vi "Append Element(s) to Dataset (Variant).vi"(4 "Data Element(s)":variant, 6 "error in (no error)":errorcluster, 8 "Dimension to Extend (0)":i32, 9 "HDF5 Dataset Ref":T1) -> (0 "error out":errorcluster, 1 "Number of Elements Added":i32, 2 "First Element Index":u64[](array[numeric]), 3 "HDF5 Dataset out":T1)   [LabVIEW 2017]
doc: "Appends one or more elements to an unlimited dataset."
uses:
  <vilib>/UPVI/lvhdf5/library.llb/HDF5 Ref.ctl
  <vilib>/UPVI/lvhdf5/error.llb/LVH5EMajorID.ctl
  <vilib>/UPVI/lvhdf5/error.llb/LVH5EMinorID.ctl
  <vilib>/UPVI/lvhdf5/dataspace.llb/H5S_seloper_t.ctl
panel:
  # "LVHDF5 Toolkit\nCopyright (c) 2005-2013 by Jason D. Sommerville\nCopyright (c) 2014 by UPVI, LLC.\n\nThis use and distribution of this file is governed by the terms found in \nLICENSE.txt distributed with this toolkit and installed at\n <user.lib>\\_lvhdf5\\LICENSE.txt"
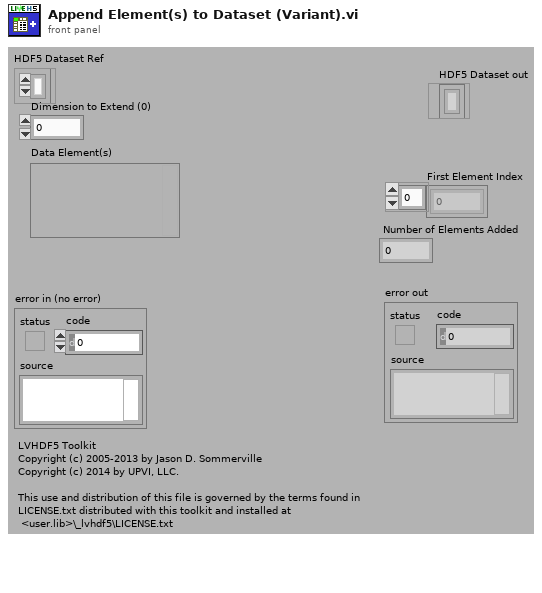
[diagram p1: front panel]
types:
  T1 = typedef "HDF5 Ref.ctl" = refnum<k1>
  T2 = typedef "LVH5EMinorID.ctl" = string
  T3 = typedef "LVH5EMajorID.ctl" = string
  T4 = typedef "H5S_seloper_t.ctl" = i32
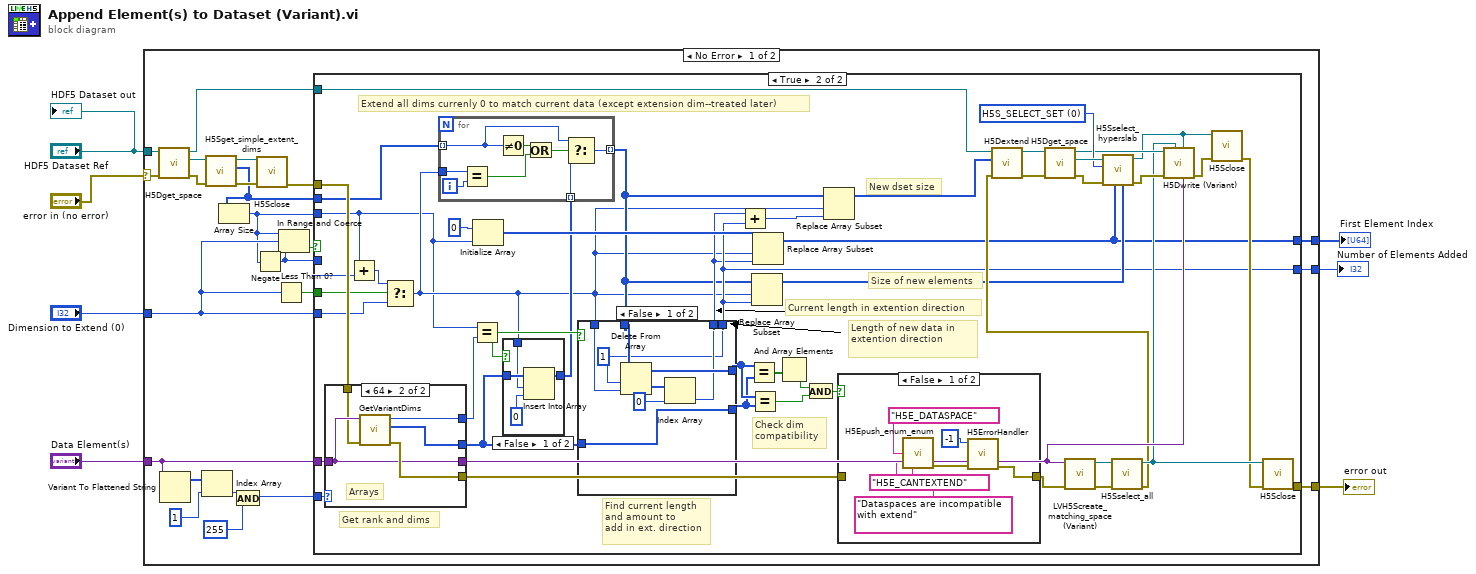
[diagram p0: block diagram]
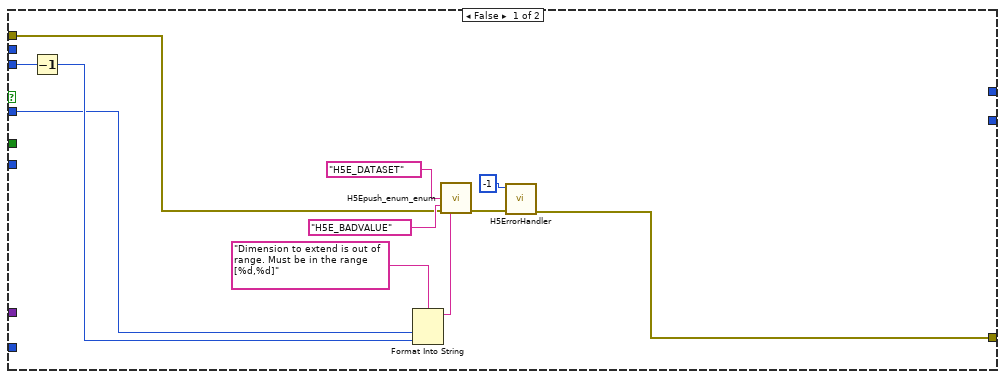
[diagram p2: hidden frame]
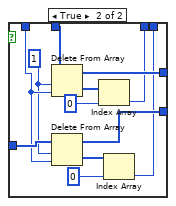
[diagram p4: hidden frame]
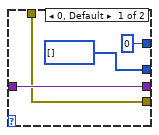
[diagram p6: hidden frame]
diagram:
  n1 = case shown="No Error" "error in (no error)" {
    selector: "error in (no error)" -> [w23 w138]
    tunnel: "HDF5 Dataset Ref" -> [w30 _]
    tunnel: "Data Element(s)" -> [w22 _]
    tunnel: [w25 w138] -> w5
    tunnel: "Dimension to Extend (0)" -> [w11 _]
    tunnel: [w16 _] -> w2
    tunnel: [w15 _] -> w1
    frame No Error {
      n2 = call <vilib>:"H5Dget_space.vi"("error in (no error)"=w23, "HDF5 Dataset Ref"=w30) -> ("error out"=w29:errorcluster, "HDF5 Dataspace Ref"=w28:T1, "HDF5 Dataset Ref out"=w12:T1)  [unwired: 5 in]
      n3 = Variant To Flattened String(Variant=w22) -> (1:w21:i16[])  [unwired: 1 out]
      n4 = Index Array(array=w21, index=1) -> (element=w18:i16)
      n5 = call <vilib>:"H5Sget_simple_extent_dims.vi"("error in (no error)"=w29, "HDF5 Space Ref"=w28) -> ("error out"=w26:errorcluster, "Dims"=w13:u64[], "HDF5 Ref out"=w27:T1)  [unwired: 4 in, 1 out]
      n6 = Array Size(array=w13) -> (size(s)=w9:i32)
      n7 = And(x=w18, y=i16 255) -> (x .and. y?=w19:i16)
      n8 = Negate(x=w9) -> (-x=w8:i32)
      n9 = call <vilib>:"H5Sclose.vi"("error in (no error)"=w26, "HDF5 Dataspace Ref"=w27) -> ("error out"=w24:errorcluster)  [unwired: 7 in]
      n10 = Less Than 0?(x=w11) -> (x < 0?=w14:bool)
      n11 = In Range and Coerce(upper limit=w9, x=w11, lower limit=w8) -> (In Range?=w10:bool)  [unwired: 1 out]
      n12 = case shown="True" w10 {
        tunnel: [w31 w75] -> w25
        tunnel: w24 -> [w37 w69]
        tunnel: w22 -> [_ w60]
        tunnel: w19 -> [_ w59]
        tunnel: [_ w56] -> w16
        tunnel: [_ w55] -> w15
        tunnel: w14 -> [_ w53]
        tunnel: w13 -> [_ w50]
        tunnel: w12 -> [_ w45]
        tunnel: w11 -> [_ w43]
        tunnel: w9 -> [w36 w42]
        tunnel: w8 -> [w33 _]
        frame False {
          n13 = Decrement(x=w36) -> (x-1=w34:i32)
          n14 = Format Into String(format string="Dimension to extend is out of range. Must be in the range [%d,%d]" ("msg"), w33, w34) -> (resulting string=w32:string)  [unwired: 2 in, 1 out]
          n15 = call <vilib>:"H5Epush_enum_enum.vi"("major_id"=T3 "H5E_DATASET", "minor_id"=T2 "H5E_BADVALUE", "error in (no error)"=w37, "msg"=w32) -> ("error out"=w38:errorcluster)  [unwired: 10 in, 1 out]
          n16 = call <vilib>:"H5ErrorHandler.vi"("error in (no error)"=w38, "herr_t"=-1) -> ("error out"=w31:errorcluster)  [unwired: 3 in, 4 out]
        }
        frame True {
          w84 = T4 0 items=["H5S_SELECT_NOOP"=-1, "H5S_SELECT_SET"=0, "H5S_SELECT_OR"=1, "H5S_SELECT_AND"=2, "H5S_SELECT_XOR"=3, "H5S_SELECT_NOTB"=4, "H5S_SELECT_NOTA"=5, "H5S_SELECT_APPEND"=6, "H5S_SELECT_PREPEND"=7] ("Operator")
          # "Extend all dims currenly 0 to match current data (except extension dim--treated later)"
          # "Find current length\nand amount to\nadd in ext. direction"
          # "Get rank and dims"
          # "Size of new elements"
          # "New dset size"
          # "Check dim\ncompatibility"
          # "Current length in extention direction"
          # "Length of new data in extention direction"
          n17 = case shown="64" w59 {
            tunnel: w60 -> [w132 w135]
            tunnel: [w129 w136] -> w66
            tunnel: [w132 w135] -> w79
            tunnel: [0 ("rank") w137] -> w51
            tunnel: [i32[] [] ("Array") w133] -> w47
            tunnel: w69 -> [w129 w134]
            frame 0, Default {
            }
            frame 64 {
              # "Arrays"
              n18 = call <vilib>:"GetVariantDims.vi"("error in (no error)"=w134, "Variant"=w135) -> ("error out"=w136:errorcluster, "Array"=w133:i32[], "rank"=w137:i32)  [unwired: 7 in]
            }
          }
          n19 = Add(x=w42, y=w43) -> (x+y=w52:i32)
          n20 = Select(t=w52, s=w53, f=w43) -> (s? t:f=w44:i32)
          n21 = Equal?(x=w42, y=w51) -> (x = y?=w48:bool)
          n22 = Initialize Array(u64 0 ("element"), w42) -> (w61:u64[])
          n23 = case shown="False" w48 {
            tunnel: w47 -> [w92 w93]
            tunnel: w44 -> [w91 _]
            tunnel: [w89 w93] -> w46
            frame False {
              n24 = Insert Into Array(array=w92, index=w91, new element=0 ("length")) -> (w89:i32[])
            }
            frame True {
            }
          }
          n25 = for {
            tunnel: w50 -> [w101] mode=indexing
            tunnel: w46 -> [w100] mode=indexing
            tunnel: [w99] -> w49 mode=indexing
            tunnel: w44 -> [w96]
            i -> [w95]
            n26 = Equal?(x=w96, y=w95) -> (x = y?=w94:bool)
            n27 = Not Equal To 0?(x=w101) -> (x != 0?=w98:bool)
            n28 = Or(x=w98, y=w94) -> (x .or. y?=w97:bool)
            n29 = Select(t=w101, s=w97, f=w100) -> (s? t:f=w99:u64)
          }
          n30 = case shown="False" w48 {
            tunnel: w49 -> [w109 w121]
            tunnel: w47 -> [w102 w116]
            tunnel: w44 -> [w104 w115]
            tunnel: [w108 w120] -> w58
            tunnel: [w102 w113] -> w57
            tunnel: [w105 w117] -> w54
            tunnel: [w103 w110] -> w56
            frame False {
              w103 = 1 ("length")
              n31 = Delete From Array(array=w109, length=w103, index=w104) -> (deleted portion=w107:u64[], array with subset deleted=w108:u64[])
              n32 = Index Array(array=w107, index=0) -> (element=w105:u64)
            }
            frame True {
              w114 = 1 ("length")
              n33 = Delete From Array(array=w121, length=w114, index=w115) -> (deleted portion=w119:u64[], array with subset deleted=w120:u64[])
              n34 = Delete From Array(array=w116, length=w114, index=w115) -> (deleted portion=w112:i32[], array with subset deleted=w113:i32[])
              n35 = Index Array(array=w119, index=0) -> (element=w117:u64)
              n36 = Index Array(array=w112, index=0) -> (element=w110:i32)
            }
          }
          n37 = Add(x=w54, y=w56) -> (x+y=w64:u64)
          n38 = Equal?(x=w58, y=w57) -> (x = y?=w73:bool[])
          n39 = Equal?(x=w58, y=w57) -> (x = y?=w71:bool)
          n40 = Replace Array Subset(array=w49, new element=w56, index=w44) -> (w63:u64[])
          n41 = Replace Array Subset(array=w61, new element=w54, index=w44) -> (w55:u64[])
          n42 = And Array Elements(Boolean array=w73) -> (logical AND=w72:bool)
          n43 = And(x=w72, y=w71) -> (x .and. y?=w70:bool)
          n44 = Replace Array Subset(array=w49, new element=w64, index=w44) -> (w65:u64[])
          n45 = case shown="False" w70 {
            tunnel: [w122 w128] -> w67
            tunnel: w66 -> [_ w128]
            frame False {
              n46 = call <vilib>:"H5Epush_enum_enum.vi"("major_id"=T3 "H5E_DATASPACE", "minor_id"=T2 "H5E_CANTEXTEND", "msg"="Dataspaces are incompatible with extend") -> ("error out"=w123:errorcluster)  [unwired: 11 in, 1 out]
              n47 = call <vilib>:"H5ErrorHandler.vi"("error in (no error)"=w123, "herr_t"=-1) -> ("error out"=w122:errorcluster)  [unwired: 3 in, 4 out]
            }
            frame True {
            }
          }
          n48 = call <vilib>:"LVH5Screate_matching_space (Variant).vi"("error in (no error)"=w67, "Data"=w79) -> ("error out"=w78:errorcluster, "HDF5 Dataspace Ref"=w77:T1)  [unwired: 6 in]
          n49 = call <vilib>:"H5Sselect_all.vi"("error in (no error)"=w78, "HDF5 Space Ref"=w77) -> ("error out"=w68:errorcluster, "HDF5 Ref out"=w76:T1)  [unwired: 6 in]
          n50 = call <vilib>:"H5Dextend.vi"("error in (no error)"=w68, "Size"=w65, "HDF5 Dataset Ref"=w45) -> ("error out"=w87:errorcluster, "HDF5 Dataset Ref out"=w88:T1)  [unwired: 5 in]
          n51 = call <vilib>:"H5Dget_space.vi"("error in (no error)"=w87, "HDF5 Dataset Ref"=w88) -> ("error out"=w86:errorcluster, "HDF5 Dataspace Ref"=w85:T1, "HDF5 Dataset Ref out"=w83:T1)  [unwired: 5 in]
          n52 = call <vilib>:"H5Sselect_hyperslab.vi"("Count"=w63, "Start"=w55, "error in (no error)"=w86, "Operator"=w84, "HDF5 Space Ref"=w85) -> ("error out"=w80:errorcluster, "HDF5 Ref out"=w82:T1)  [unwired: 5 in]
          n53 = call <vilib>:"H5Dwrite (Variant).vi"("Data"=w79, "HDF5 File Space Ref (H5S_ALL)"=w82, "HDF5 Memory Space Ref (H5S_ALL)"=w76, "error in (no error)"=w80, "HDF5 Dataset Ref"=w83) -> ("error out"=w81:errorcluster)  [unwired: 5 in, 1 out]
          n54 = call <vilib>:"H5Sclose.vi"("error in (no error)"=w81, "HDF5 Dataspace Ref"=w82) -> ("error out"=w74:errorcluster)  [unwired: 7 in]
          n55 = call <vilib>:"H5Sclose.vi"("error in (no error)"=w74, "HDF5 Dataspace Ref"=w76) -> ("error out"=w75:errorcluster)  [unwired: 7 in]
        }
      }
    }
    frame Error {
    }
  }
  "error out" <- w5
  "Number of Elements Added" <- w2
  "First Element Index" <- w1
  "HDF5 Dataset out" <- "HDF5 Dataset Ref"
